vi "Module Type.vi"(11 "System Health Module in":refnum<class "System Health Module.lvclass">) -> (2 "Module Type":string)   [LabVIEW 2020, in "Volatus.lvlib" / "System Health Module.lvclass"]
uses:
  System Health Module.lvclass
  System Health Module.lvclass/System Health Module.ctl
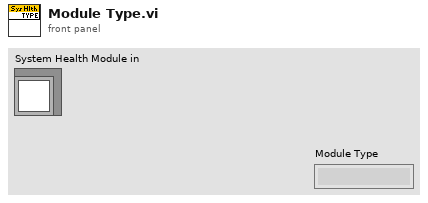
[diagram p1: front panel]
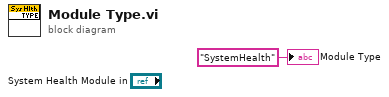
[diagram p0: block diagram]
diagram:
  "Module Type" <- "SystemHealth" ("Module Type")
